vi "Write Generated Files.vi"(8 "error in (no error)":errorcluster, 10 "Generated Files":path[](array[path]), 11 "Task Outputs in":refnum<class "Task Outputs.lvclass">) -> (0 "error out":errorcluster, 3 "Task Outputs out":refnum<class "Task Outputs.lvclass">)   [LabVIEW 2017, in "Message Interface.lvlib" / "Task Outputs.lvclass"]
uses:
  Task Outputs.lvclass
  Task Outputs.lvclass/Task Outputs.ctl
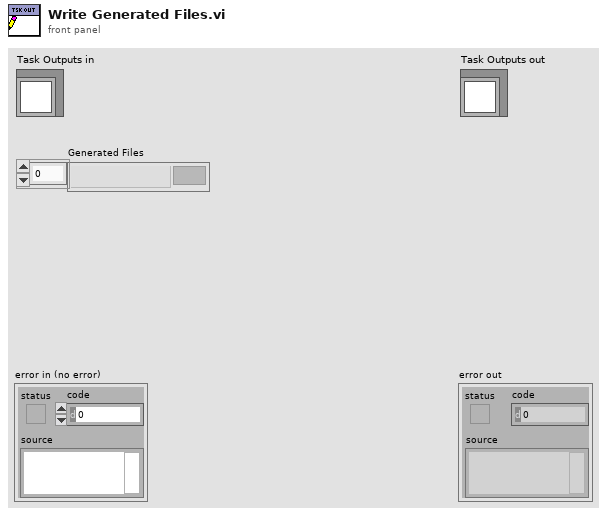
[diagram p1: front panel]
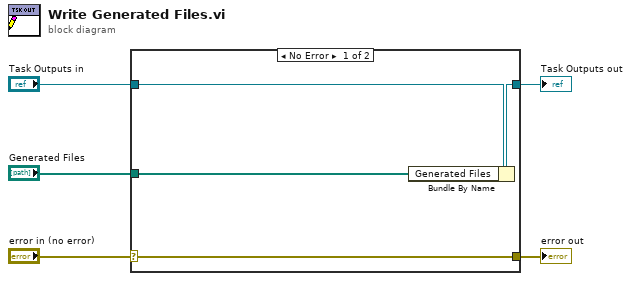
[diagram p0: block diagram]
diagram:
  n1 = case shown="No Error" "error in (no error)" {
    selector: "error in (no error)" -> [w9 w10]
    tunnel: [w9 w10] -> w4
    tunnel: [w7 w11] -> w2
    tunnel: "Task Outputs in" -> [w8 w11]
    tunnel: "Generated Files" -> [w6 _]
    frame No Error {
      n2 = Bundle By Name(cluster=w8, "Generated Files"=w6) -> (w7:refnum<class "Task Outputs.lvclass">)
    }
    frame Error {
    }
  }
  "error out" <- w4
  "Task Outputs out" <- w2
